vi "Inputs.vi"(8 "error in (no error)":errorcluster, 11 "State in":T1={"State"=enum."Idle", "Start Time"=timestamp(0 s since 1904-01-01), "Configuration"={"Cycle Period"=0.0, "Ismatech"={"VISA resource name"="", "Simulated?"=FALSE, "Pump Number"=1.0, "Reverse?"=FALSE}, "Masterflex"={"VISA resource name"="", "Simulated?"=FALSE, "Pump Number"=1.0, "Reverse?"=FALSE}, "Mettler"={"VISA resource name"="", "Simulated?"=FALSE}, "Bronkhorst M13 Flow Meter"={"VISA resource name"="", "Simulated?"=FALSE}, "PID 2 Parameters"={"Input Device"=enum."Bronkhorst M13", "Output Device"=enum."Ismatec ISM 831C", "Setpoint"=0.0, "PID gains"={"proportional gain (Kc)"=1.0, "integral time (Ti, min)"=0.01, "derivative time (Td, min)"=0.0}}, "Manual Entry"=0.0, "Auto?"=TRUE, "output range"={"output high"=100.0, "output low"=0.0}, "Bronkhorst M14"={"VISA resource name"="", "Simulated?"=FALSE}, "Tacmina Settings"={"Analog DAQ Task"="", "Digital DAQ Task"=""}, "KNF SIMDOS Settings"={"VISA resource name"="", "Simulated?"=TRUE}, "ASIA Pump C"={"ASIA Pump #"=0, "channel"=0, "Simulated"=FALSE}, "VICI Settings"={"VISA resource name"="", "Simulated?"=FALSE, "Pump Letter"="", "Reverse?"=FALSE}, "FLOM Settings"={"VISA resource name"="", "Simulated?"=TRUE, "Pump Number"=0.0}, "SSI PR Settings"={"VISA resource name"="", "Simulated?"=FALSE}}, "Current Time"=timestamp(0 s since 1904-01-01), "PID 1 Parameters"={"Setpoint"=0.0, "PID gains"={"proportional gain (Kc)"=1.0, "integral time (Ti, min)"=0.01, "derivative time (Td, min)"=0.0}}, "First Iteration"=FALSE, "Data"={"Flowmeter Output"=0.0, "Density"=0.0, "FL Temp"=0.0, "Scale Output (g)"=0.0, "Scale Rate of Change (g/min)"=0.0, "PID 1 Output"=0.0, "PID 2 Process Variable"=0.0, "PID 2 output"=0.0, "Pump Flow"=0.0, "Pump Pressure"=0.0}, "Process Name"="", "Pump On?"=enum."Off", "Input Error"=FALSE, "Output Error"=FALSE, "Log Started"=FALSE, "Current Setpoint"=0.0} {"PID 1 Parameters"."PID gains"."derivative time (Td, min)" format="%.3f"; "PID 1 Parameters"."PID gains"."integral time (Ti, min)" format="%.3f"; "PID 1 Parameters"."PID gains"."proportional gain (Kc)" format="%.3f"; "Configuration"."output range"."output low" min=0.0 max=100.0 format="%.2f"; "Configuration"."output range"."output high" format="%.2f"; "Configuration"."PID 2 Parameters"."PID gains"."derivative time (Td, min)" format="%.3f"; "Configuration"."PID 2 Parameters"."PID gains"."integral time (Ti, min)" format="%.3f"; "Configuration"."PID 2 Parameters"."PID gains"."proportional gain (Kc)" format="%.3f"; "Configuration"."ASIA Pump C"."channel" min=0 max=1 step=1; "Configuration"."Ismatech"."Pump Number" min=1.0 max=20.0 step=1.0; "Configuration"."Masterflex"."Pump Number" min=1.0 max=20.0 step=1.0}) -> (0 "error out":errorcluster, 3 "State out":T1={"State"=enum."Idle", "Start Time"=timestamp(0 s since 1904-01-01), "Configuration"={"Cycle Period"=0.0, "Ismatech"={"VISA resource name"="", "Simulated?"=FALSE, "Pump Number"=1.0, "Reverse?"=FALSE}, "Masterflex"={"VISA resource name"="", "Simulated?"=FALSE, "Pump Number"=1.0, "Reverse?"=FALSE}, "Mettler"={"VISA resource name"="", "Simulated?"=FALSE}, "Bronkhorst M13 Flow Meter"={"VISA resource name"="", "Simulated?"=FALSE}, "PID 2 Parameters"={"Input Device"=enum."Bronkhorst M13", "Output Device"=enum."Ismatec ISM 831C", "Setpoint"=0.0, "PID gains"={"proportional gain (Kc)"=1.0, "integral time (Ti, min)"=0.01, "derivative time (Td, min)"=0.0}}, "Manual Entry"=0.0, "Auto?"=TRUE, "output range"={"output high"=100.0, "output low"=0.0}, "Bronkhorst M14"={"VISA resource name"="", "Simulated?"=FALSE}, "Tacmina Settings"={"Analog DAQ Task"="", "Digital DAQ Task"=""}, "KNF SIMDOS Settings"={"VISA resource name"="", "Simulated?"=TRUE}, "ASIA Pump C"={"ASIA Pump #"=0, "channel"=0, "Simulated"=FALSE}, "VICI Settings"={"VISA resource name"="", "Simulated?"=FALSE, "Pump Letter"="", "Reverse?"=FALSE}, "FLOM Settings"={"VISA resource name"="", "Simulated?"=TRUE, "Pump Number"=0.0}, "SSI PR Settings"={"VISA resource name"="", "Simulated?"=FALSE}}, "Current Time"=timestamp(0 s since 1904-01-01), "PID 1 Parameters"={"Setpoint"=0.0, "PID gains"={"proportional gain (Kc)"=1.0, "integral time (Ti, min)"=0.01, "derivative time (Td, min)"=0.0}}, "First Iteration"=FALSE, "Data"={"Flowmeter Output"=0.0, "Density"=0.0, "FL Temp"=0.0, "Scale Output (g)"=0.0, "Scale Rate of Change (g/min)"=0.0, "PID 1 Output"=0.0, "PID 2 Process Variable"=0.0, "PID 2 output"=0.0, "Pump Flow"=0.0, "Pump Pressure"=0.0}, "Process Name"="", "Pump On?"=enum."Off", "Input Error"=FALSE, "Output Error"=FALSE, "Log Started"=FALSE, "Current Setpoint"=0.0} {"PID 1 Parameters"."PID gains"."derivative time (Td, min)" format="%.3f"; "PID 1 Parameters"."PID gains"."integral time (Ti, min)" format="%.3f"; "PID 1 Parameters"."PID gains"."proportional gain (Kc)" format="%.3f"; "Configuration"."output range"."output low" min=0.0 max=100.0 format="%.2f"; "Configuration"."output range"."output high" format="%.2f"; "Configuration"."PID 2 Parameters"."PID gains"."derivative time (Td, min)" format="%.3f"; "Configuration"."PID 2 Parameters"."PID gains"."integral time (Ti, min)" format="%.3f"; "Configuration"."PID 2 Parameters"."PID gains"."proportional gain (Kc)" format="%.3f"; "Configuration"."ASIA Pump C"."channel" min=0 max=1 step=1; "Configuration"."Ismatech"."Pump Number" min=1.0 max=20.0 step=1.0; "Configuration"."Masterflex"."Pump Number" min=1.0 max=20.0 step=1.0})   [LabVIEW 2018, in "Feed Module.lvlib" / "Feed Module Engine.lvlib"]
uses:
  Feed Module Engine.lvlib
  State Cluster.ctl
  State Enum.ctl
  Feed Module/Controls/Feed Module Settings Cluster.ctl
  Ismatec ISM 831C/Controls/Ismatech Settings Cluster.ctl
  Masterflex 7550-30/Controls/Settings Cluster.ctl
  Mettler Toledo/Controls/Settings Cluster.ctl
  Bronkhorst M13 Flow Meter/Settings Cluster.ctl
  PID 2 Parameters Cluster.ctl
  PID Input Enum.ctl
  PID 2 Output Enum.ctl
  Tacmina QI/Tacmina QI DAQ Setting.ctl
  KNF Pump/Settings Cluster plus SIMDOS.ctl
  ASIA Pump/Pump Settings.ctl
  VICI M50 Party Mode/Settings Cluster.ctl
  FLOM Pump/Settings Cluster.ctl
  SSI PR Class/SSI PR Settings Cluster.ctl
  PID 1 Parameters Cluster.ctl
  Tag VIs/Tag FGV Operation Enum.ctl
  Mettler Toledo/Mettler Toledo.lvlib
  Bronkhorst M13 Flow Meter/Bronkhorst M13 Flow Meter.lvlib
  Shared Variables/Dynamic Shared Variables.lvlib
  Bronkhorst M14 Flow Meter/Bronkhorst M14 Flow Meter.lvlib
  Feed Module/Feed Module.lvlib
  Ismatec ISM 831C/Ismatec ISM 831C.lvlib
  Masterflex 7550-30/Masterflex 7550-30.lvlib
  Tacmina QI/Tacmina QI.lvlib
  KNF Pump/KNF SIMDOS.lvlib
  ASIA Pump.lvlib
  VICI M50 Party Mode/VICI M50 Party Mode.lvlib
  FLOM Pump/FLOM Pump.lvlib
  SSI PR Class/SSI PR Pump.lvlib
panel:
  # "Output Instruments"
  # "Input Instruments"
  # "Output Instruments"
  # "Input Instruments"
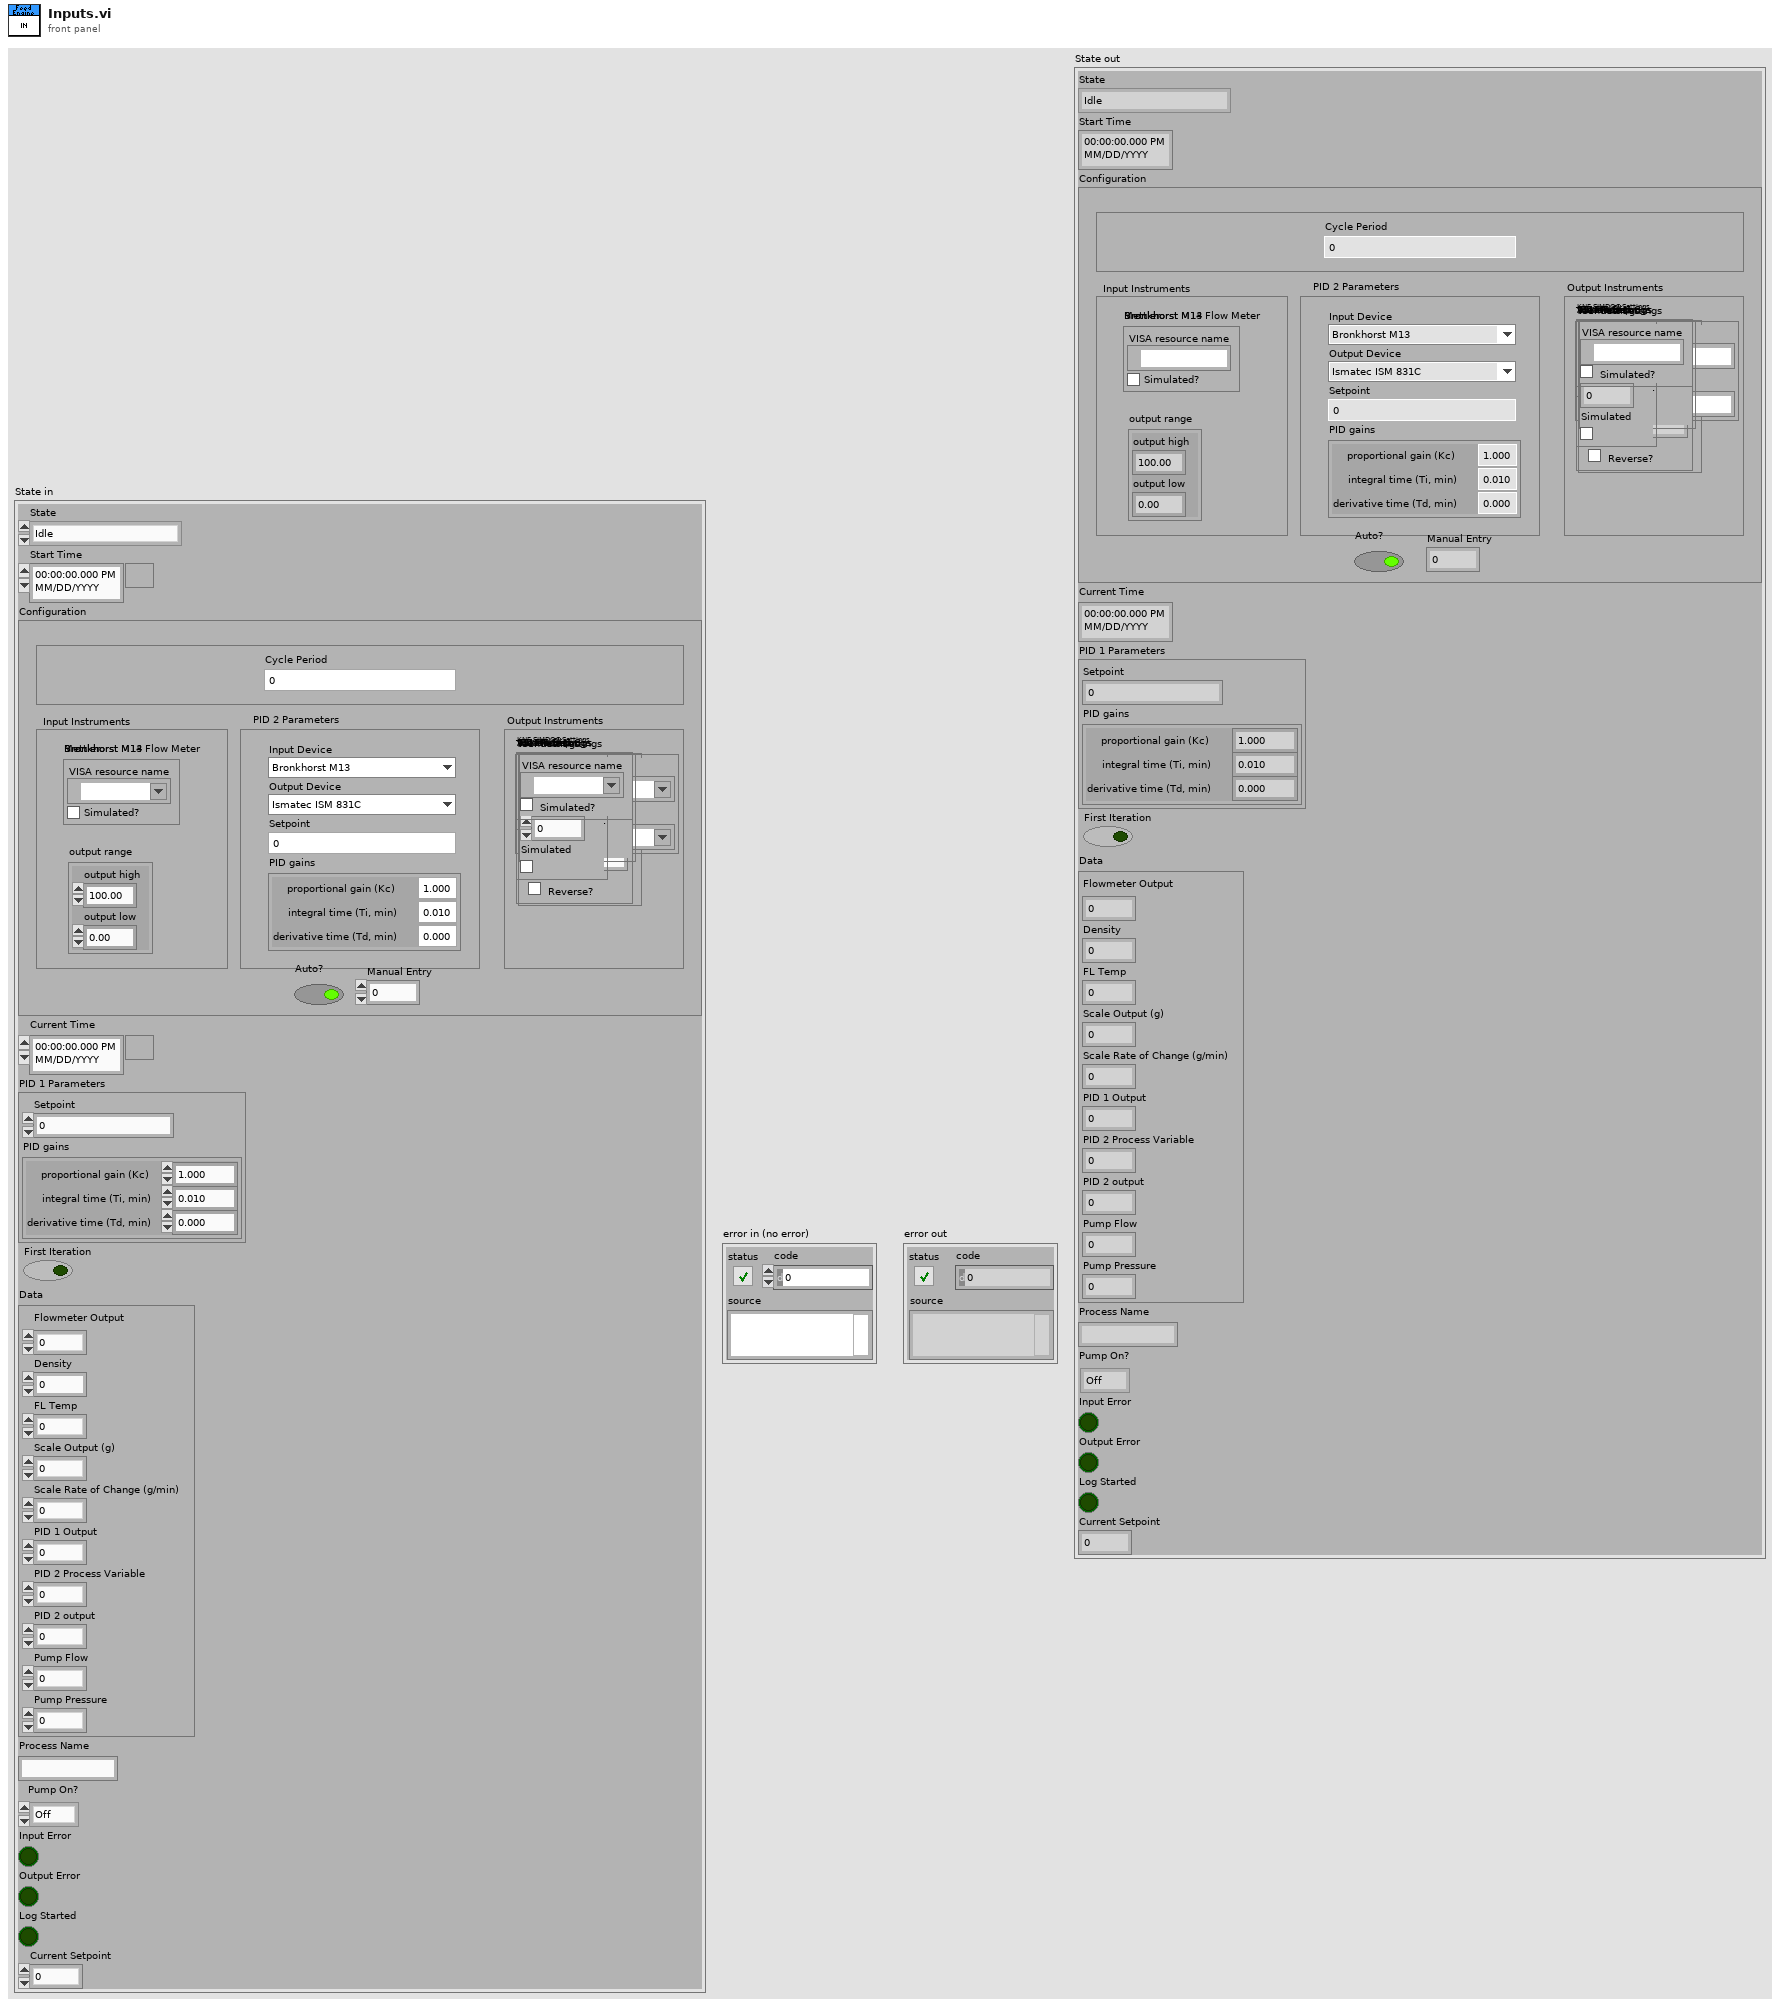
[diagram p1: front panel]
types:
  T1 = typedef "Feed Module.lvlib/Feed Module Engine.lvlib/State Cluster.ctl" = cluster{"State":T2, "Start Time":timestamp, "Configuration":T3, "Current Time":timestamp, "PID 1 Parameters":T17, "First Iteration":bool, "Data":cluster{"Flowmeter Output":dbl, "Density":dbl, "FL Temp":dbl, "Scale Output (g)":dbl, "Scale Rate of Change (g/min)":dbl, "PID 1 Output":dbl, "PID 2 Process Variable":dbl, "PID 2 output":dbl, "Pump Flow":dbl, "Pump Pressure":dbl}, "Process Name":string, "Pump On?":enum16{"Off", "On", "Not Initialized"}, "Input Error":bool, "Output Error":bool, "Log Started":bool, "Current Setpoint":dbl}
  T2 = typedef "Feed Module.lvlib/Feed Module Engine.lvlib/State Enum.ctl" = enum16{"Measuring", "Idle", "Paused"}
  T3 = typedef "Feed Module.lvlib/Feed Module Settings Cluster.ctl" = cluster{"Cycle Period":dbl, "Ismatech":T4, "Masterflex":T5, "Mettler":T6, "Bronkhorst M13 Flow Meter":T7, "PID 2 Parameters":T8, "Manual Entry":dbl, "Auto?":bool, "output range":cluster{"output high":dbl, "output low":dbl}, "Bronkhorst M14":T6, "Tacmina Settings":T11, "KNF SIMDOS Settings":T12, "ASIA Pump C":T13, "VICI Settings":T14, "FLOM Settings":T15, "SSI PR Settings":T16}
  T4 = typedef "Ismatec ISM 831C.lvlib/Ismatech Settings Cluster.ctl" = cluster{"VISA resource name":refnum<visa-resource-name>, "Simulated?":bool, "Pump Number":dbl, "Reverse?":bool}
  T5 = typedef "Masterflex 7550-30.lvlib/Settings Cluster.ctl" = cluster{"VISA resource name":refnum<visa-resource-name>, "Simulated?":bool, "Pump Number":dbl, "Reverse?":bool}
  T6 = typedef "Mettler Toledo.lvlib/Settings Cluster.ctl" = cluster{"VISA resource name":refnum<visa-resource-name>, "Simulated?":bool}
  T7 = typedef "Bronkhorst M13 Flow Meter.lvlib/Settings Cluster.ctl" = cluster{"VISA resource name":refnum<visa-resource-name>, "Simulated?":bool}
  T8 = typedef "PID 2 Parameters Cluster.ctl" = cluster{"Input Device":T9, "Output Device":T10, "Setpoint":dbl, "PID gains":cluster{"proportional gain (Kc)":dbl, "integral time (Ti, min)":dbl, "derivative time (Td, min)":dbl}}
  T9 = typedef "PID Input Enum.ctl" = enum16{"Default", "Bronkhorst M13", "Bronkhorst M14", "Scale Rate of Change"}
  T10 = typedef "PID 2 Output Enum.ctl" = enum16{"Default", "Ismatec ISM 831C", "Masterflex 7550-30", "VICI", "Tacmina QI", "KNF SIMDOS", "ASIA Type C", "FLOM UI-22-11", "SSI PR"}
  T11 = typedef "Tacmina QI.lvlib/Tacmina QI DAQ Setting.ctl" = cluster{"Analog DAQ Task":refnum<k21>, "Digital DAQ Task":refnum<k21>}
  T12 = typedef "KNF SIMDOS.lvlib/Settings Cluster plus SIMDOS.ctl" = cluster{"VISA resource name":refnum<visa-resource-name>, "Simulated?":bool}
  T13 = typedef "ASIA Pump.lvlib/Pump Settings.ctl" = cluster{"ASIA Pump #":i32, "channel":i32, "Simulated":bool}
  T14 = typedef "VICI M50 Party Mode.lvlib/Settings Cluster.ctl" = cluster{"VISA resource name":refnum<visa-resource-name>, "Simulated?":bool, "Pump Letter":string, "Reverse?":bool}
  T15 = typedef "FLOM Pump.lvlib/Settings Cluster.ctl" = cluster{"VISA resource name":refnum<visa-resource-name>, "Simulated?":bool, "Pump Number":dbl}
  T16 = typedef "SSI PR Pump.lvlib/SSI PR Settings Cluster.ctl" = cluster{"VISA resource name":refnum<visa-resource-name>, "Simulated?":bool}
  T17 = typedef "PID 1 Parameters Cluster.ctl" = cluster{"Setpoint":dbl, "PID gains":cluster{"proportional gain (Kc)":dbl, "integral time (Ti, min)":dbl, "derivative time (Td, min)":dbl}}
  T18 = typedef "Tag FGV Operation Enum.ctl" = enum16{"Init", "Set Notification Queue", "Create Tag", "Commit", "Write Tag (Numeric)", "Write Tag (Boolean)", "Read All Tags", "Read One Tag", "Delete Tag Category", "Set Alarm Parameters (Numeric)", "Set Alarm Parameters (Boolean)", "Enable All Alarms", "Disable All Alarms", "Delete All Tags", "Read Alarms", "Ack Alarm"}
  T19 = typedef "Bronkhorst M14 Flow Meter.lvlib/Settings Cluster.ctl" = cluster{"VISA resource name":refnum<visa-resource-name>, "Simulated?":bool}
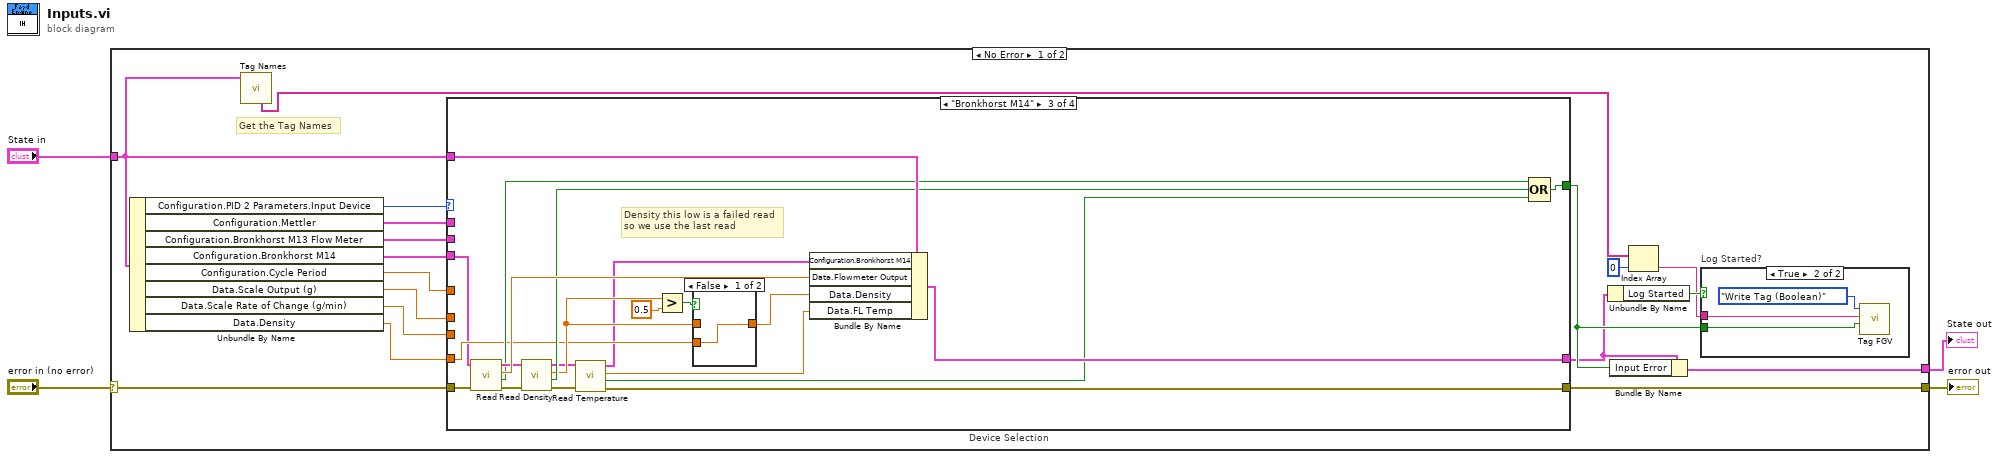
[diagram p0: block diagram]
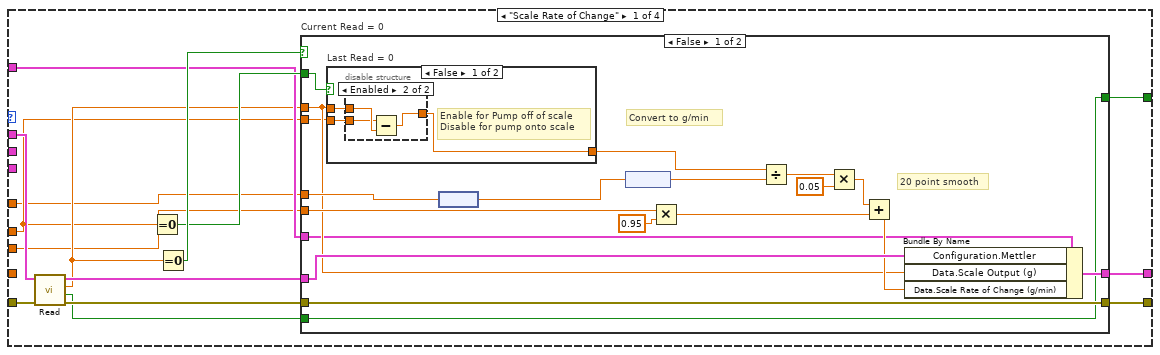
[diagram p3: hidden frame]
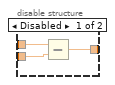
[diagram p4: hidden frame]
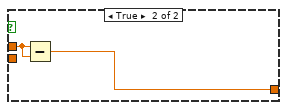
[diagram p5: hidden frame]
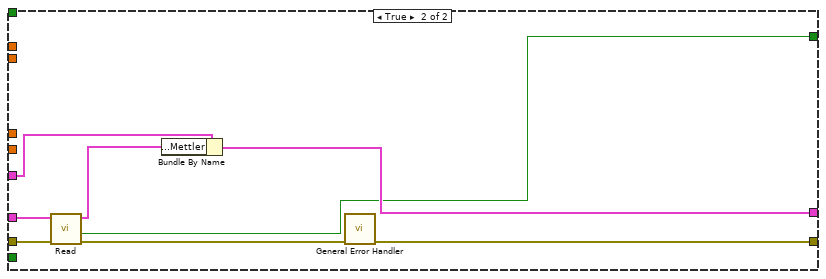
[diagram p6: hidden frame]
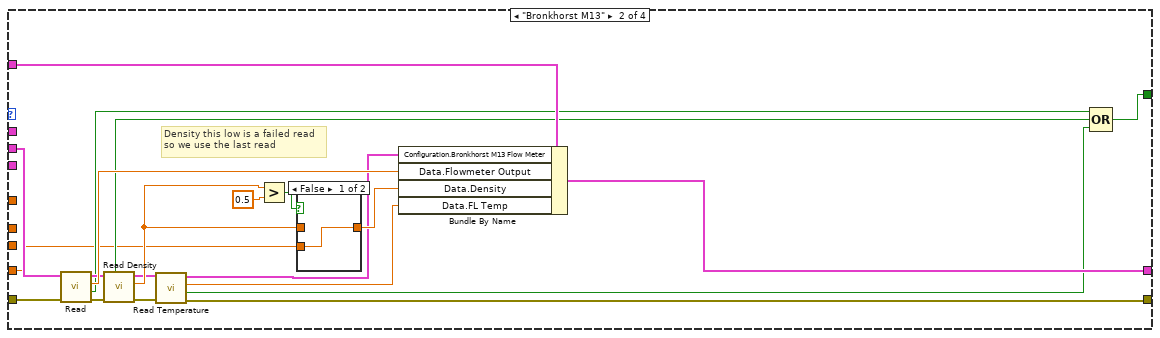
[diagram p7: hidden frame]
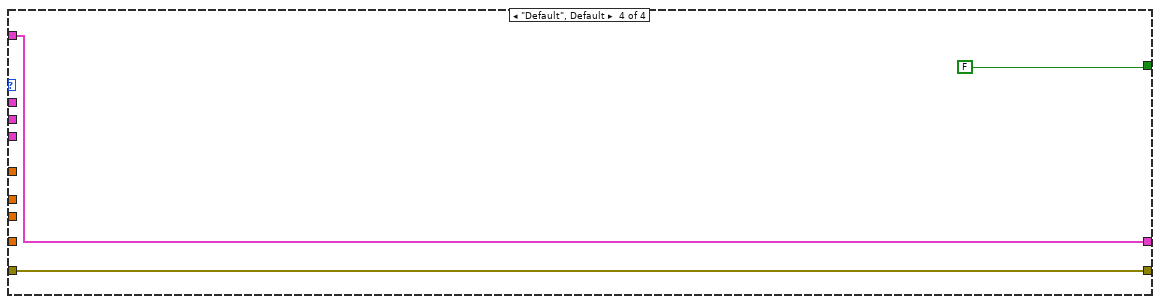
[diagram p10: hidden frame]
diagram:
  n1 = case shown="No Error" "error in (no error)" {
    selector: "error in (no error)" -> [w19 w128]
    tunnel: [w16 w128] -> w1
    tunnel: "State in" -> [w10 w127]
    tunnel: [w14 w127] -> w2
    frame No Error {
      # "Get the Tag Names"
      n2 = Unbundle By Name(w10) -> ("Configuration.PID 2 Parameters.Input Device"=w22:T9, "Configuration.Mettler"=w21:T6, "Configuration.Bronkhorst M13 Flow Meter"=w20:T7, "Configuration.Bronkhorst M14"=w8:T6, "Configuration.Cycle Period"=w9:dbl, "Data.Scale Output (g)"=w18:dbl, "Data.Scale Rate of Change (g/min)"=w17:dbl, "Data.Density"=w13:dbl)
      n3 = call "Tag Names.vi"("State in"=w10) -> ("All Boolean Tags"=w7:string[])  [unwired: 6 in, 4 out]
      n4 = case "Device Selection" shown="\"Bronkhorst M14\"" w22 {
        tunnel: w10 -> [w35 w98 w121 w126]
        tunnel: [w31 w97 w120 w126] -> w12
        tunnel: w21 -> [w39 _ _ _]
        tunnel: w20 -> [_ w94 _ _]
        tunnel: w9 -> [w32 _ _ _]
        tunnel: w19 -> [w40 w95 w118 w125]
        tunnel: [w29 w80 w104 w125] -> w16
        tunnel: w18 -> [w33 _ _ _]
        tunnel: w17 -> [w28 _ _ _]
        tunnel: [w27 w89 w113 FALSE ("Connection Error")] -> w15
        tunnel: w13 -> [_ w84 w108 _]
        tunnel: w8 -> [_ _ w101 _]
        frame "Scale Rate of Change" {
          n5 = call "Read.vi"("error in (no error)"=w40, "Mettler Settings in"=w39) -> ("error out"=w30:errorcluster, "Connection Error"=w26:bool, "mass (g)"=w34:dbl, "Mettler Settings out"=w36:T6)  [unwired: 6 in]
          n6 = Equal To 0?(x=w33) -> (x = 0?=w37:bool)
          n7 = Equal To 0?(x=w34) -> (x = 0?=w38:bool)
          n8 = case "Current Read = 0" shown="False" w38 {
            tunnel: w34 -> [w44 _]
            tunnel: w33 -> [w43 _]
            tunnel: w35 -> [w41 w74]
            tunnel: w36 -> [w59 w77]
            tunnel: [w58 w72] -> w31
            tunnel: w32 -> [w55 _]
            tunnel: w37 -> [w53 _]
            tunnel: w30 -> [w52 w75]
            tunnel: [w52 w73] -> w29
            tunnel: w28 -> [w45 _]
            tunnel: [w42 w71] -> w27
            tunnel: w26 -> [w42 _]
            frame False {
              # "20 point smooth"
              # "Convert to g/min"
              n9 = case "Last Read = 0" shown="False" w53 {
                tunnel: [w61 w70] -> w57
                tunnel: w44 -> [w60 w69]
                tunnel: w43 -> [w62 _]
                frame False {
                  # "Enable for Pump off of scale\nDisable for pump onto scale"
                  n10 = disable-structure shown="Enabled" {
                    disable-tunnel: w62 -> [w65 w67]
                    disable-tunnel: w60 -> [w64 w68]
                    disable-tunnel: [w63 w66] -> w61
                    frame Disabled {
                      n11 = Subtract(x=w64, y=w65) -> (x-y=w63:dbl)
                    }
                    frame Enabled {
                      n12 = Subtract(x=w67, y=w68) -> (x-y=w66:dbl)
                    }
                  }
                }
                frame True {
                  n13 = Subtract(x=w69, y=w69) -> (x-y=w70:dbl)
                }
              }
              n14 = node(w55) -> (w54:dbl[unit])
              n15 = node(w54) -> (w56:dbl)
              n16 = Multiply(x=w45, y=0.95) -> (x*y=w51:dbl)
              n17 = Divide(x=w57, y=w56) -> (x/y=w47:dbl)
              n18 = Multiply(x=w47, y=0.05) -> (x*y=w48:dbl)
              n19 = Add(x=w48, y=w51) -> (x+y=w46:dbl)
              n20 = Bundle By Name(cluster=w41, "Configuration.Mettler"=w59, "Data.Scale Output (g)"=w44, "Data.Scale Rate of Change (g/min)"=w46) -> (w58:T1)
            }
            frame True {
              n21 = call "Read.vi"("error in (no error)"=w75, "Mettler Settings in"=w77) -> ("error out"=w73:errorcluster, "Connection Error"=w71:bool, "Mettler Settings out"=w76:T6)  [unwired: 6 in, 1 out]
              n22 = Bundle By Name(cluster=w74, "Configuration.Mettler"=w76) -> (w72:T1)
              n23 = call <vilib>:"General Error Handler.vi"("error in (no error)"=w73) -> ()  [unwired: 10 in, 5 out]
            }
          }
        }
        frame "Bronkhorst M13" {
          # "Density this low is a failed read\nso we use the last read"
          n24 = call "Read.vi"("error in (no error)"=w95, "Bronkhorst Settings in"=w94) -> ("error out"=w93:errorcluster, "Connection Error"=w91:bool, "flow"=w96:dbl, "Bronkhorst Settings out"=w92:T7)  [unwired: 6 in]
          n25 = call "Read Density.vi"("error in (no error)"=w93, "Bronkhorst Settings in"=w92) -> ("error out"=w83:errorcluster, "Connection Error"=w90:bool, "Density kg/m^3"=w86:sgl, "Bronkhorst Settings out"=w82:T7)  [unwired: 6 in]
          n26 = call "Read Temperature.vi"("error in (no error)"=w83, "Bronkhorst Settings in"=w82) -> ("error out"=w80:errorcluster, "Connection Error"=w78:bool, "Temp (C)"=w79:sgl, "Bronkhorst Settings out"=w81:T7)  [unwired: 6 in]
          n27 = Greater?(x=w86, y=sgl 0.5) -> (0:w88:bool)
          n28 = case shown="False" w88 {
            tunnel: w86 -> [_ w100]
            tunnel: [w99 w100] -> w85
            tunnel: w84 -> [w99 _]
            frame False {
            }
            frame True {
            }
          }
          n29 = Bundle By Name(cluster=w98, "Configuration.Bronkhorst M13 Flow Meter"=w81, "Data.Flowmeter Output"=w96, "Data.Density"=w85, "Data.FL Temp"=w79) -> (w97:T1)
          n30 = Compound Arithmetic op=OR(w91, w90, w78) -> (w89:bool)
        }
        frame "Bronkhorst M14" {
          # "Density this low is a failed read\nso we use the last read"
          n31 = call "Read.vi"("error in (no error)"=w118, "Bronkhorst Settings in"=w101) -> ("error out"=w117:errorcluster, "Connection Error"=w115:bool, "flow"=w119:dbl, "Bronkhorst Settings out"=w116:T19)  [unwired: 6 in]
          n32 = call "Read Density.vi"("error in (no error)"=w117, "Bronkhorst Settings in"=w116) -> ("error out"=w107:errorcluster, "Connection Error"=w114:bool, "Density kg/m^3"=w110:sgl, "Bronkhorst Settings out"=w106:T7)  [unwired: 6 in]
          n33 = call "Read Temperature.vi"("error in (no error)"=w107, "Bronkhorst Settings in"=w106) -> ("error out"=w104:errorcluster, "Connection Error"=w102:bool, "Temp (C)"=w103:sgl, "Bronkhorst Settings out"=w105:T7)  [unwired: 6 in]
          n34 = Greater?(x=w110, y=sgl 0.5) -> (0:w112:bool)
          n35 = case shown="False" w112 {
            tunnel: w110 -> [_ w123]
            tunnel: [w122 w123] -> w109
            tunnel: w108 -> [w122 _]
            frame False {
            }
            frame True {
            }
          }
          n36 = Bundle By Name(cluster=w121, "Configuration.Bronkhorst M14"=w105, "Data.Flowmeter Output"=w119, "Data.Density"=w109, "Data.FL Temp"=w103) -> (w120:T1)
          n37 = Compound Arithmetic op=OR(w115, w114, w102) -> (w113:bool)
        }
        frame "Default", Default {
        }
      }
      n38 = Unbundle By Name(w12) -> ("Log Started"=w11:bool)
      n39 = Bundle By Name(cluster=w12, "Input Error"=w15) -> (w14:T1)
      n40 = Index Array(array=w7, index=0) -> (element=w5:string)
      n41 = case "Log Started?" shown="True" w11 {
        tunnel: w5 -> [_ w25]
        tunnel: w15 -> [_ w23]
        frame False {
        }
        frame True {
          n42 = call "Tag FGV.vi"("Data"=w23, "Tag Name"=w25, "Operation"=Tag_FGV_Operation_Enum."Write Tag (Boolean)") -> ()  [unwired: 3 in, 6 out]
        }
      }
    }
    frame Error {
    }
  }
  "error out" <- w1
  "State out" <- w2
